vi "E1A_Waveform.vi"(11 "Data in":dbl[](array[numeric])) -> (3 "WF out":waveform(dbl)[](array[waveform]))   [LabVIEW 2022 SP3]
panel:
  out "appended array":dbl[](array[numeric])
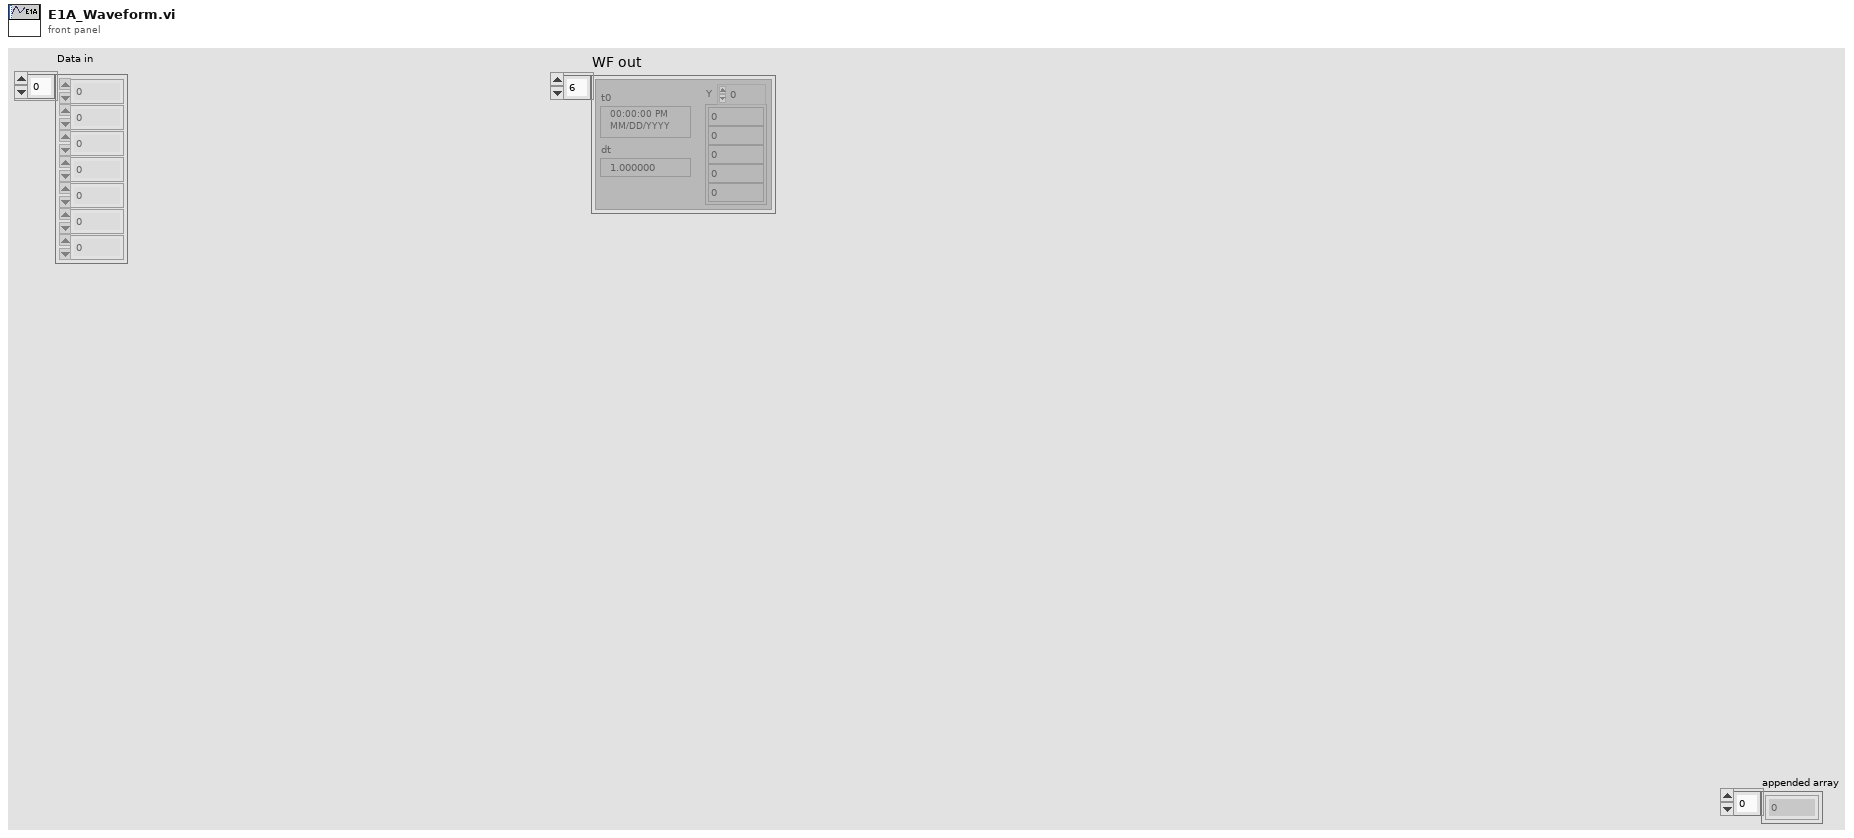
[diagram p1: front panel]
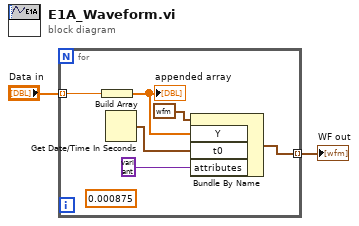
[diagram p0: block diagram]
diagram:
  n1 = for {
    tunnel: "Data in" -> [w5] mode=indexing
    tunnel: [w7] -> w2 mode=indexing
    (unwired) 0.000875 ("dt")
    n2 = Build Array(w5) -> (w4:dbl[])
    "appended array" <- w4
    n3 = Get Date/Time In Seconds() -> (seconds since 1Jan1904=w3:timestamp)
    n4 = Bundle By Name(cluster=waveform(dbl) {"t0"=timestamp(0 s since 1904-01-01), "dt"=1.0, "Y"=[]} ("waveform"), "Y"=w4, "t0"=w3, "attributes"=variant) -> (w7:waveform(dbl))
  }
  "WF out" <- w2
